vi "SelectOPCTags.RecurseThroughCurrent.vi"(8 "error in (no error)":errorcluster, 9 "Parent":string, 10 "Node Pointer":u64[](array[numeric]) format="%.0x", 11 "Tree":refnum<vi>) -> (0 "error out":errorcluster, 3 "Tree Out":refnum<vi>)   [LabVIEW 2019, in "OPC UA Client Addon System Explorer.lvlib"]
uses:
  OPC UA Client Addon System Explorer.lvlib
  <vilib>/NI VeriStand/Custom Device API/Custom Device API.lvlib
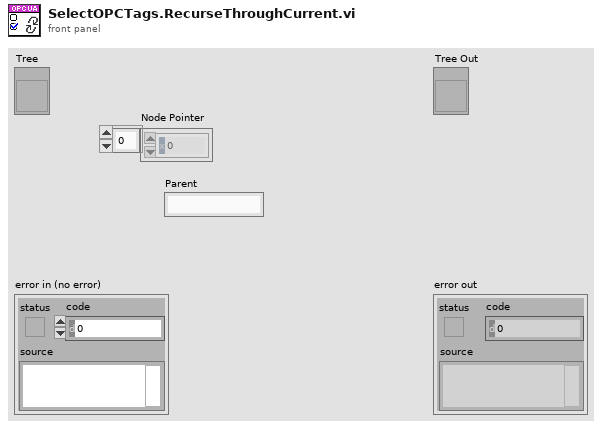
[diagram p1: front panel]
types:
  T1 = typedef "Custom Device API.lvlib/Custom Device Item Info.ctl" = cluster{"Name":string, "Is Channel":bool, "GUID":string, "Is Waveform":bool}
  T2 = typedef "Custom Device API.lvlib/Custom Device Item Ref.ctl" = u64
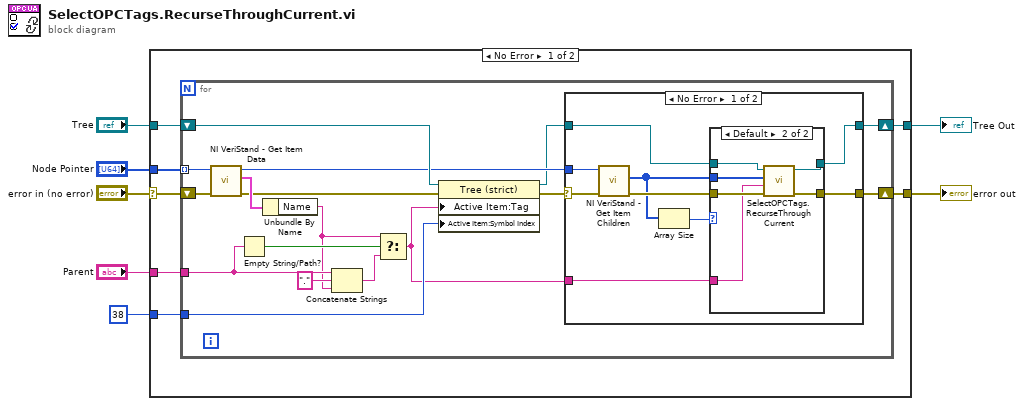
[diagram p0: block diagram]
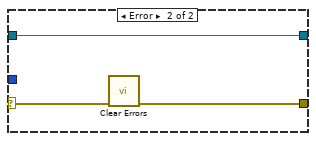
[diagram p3: hidden frame]
diagram:
  n1 = case shown="No Error" "error in (no error)" {
    selector: "error in (no error)" -> [w14 w53]
    tunnel: [w13 w53] -> w6
    tunnel: "Tree" -> [w11 w52]
    tunnel: [w12 w52] -> w4
    tunnel: 38 ("Symbol Index (38)") -> [w10 _]
    tunnel: "Node Pointer" -> [w9 _]
    tunnel: "Parent" -> [w8 _]
    frame No Error {
      n2 = for {
        tunnel: w10 -> [w30]
        shift-right: [w23] -> w13
        shift-left: w14 -> [w29]
        shift-right: [w21] -> w12
        shift-left: w11 -> [w31]
        tunnel: w9 -> [w28] mode=indexing
        tunnel: w8 -> [w20]
        n3 = call <vilib>:"NI VeriStand - Get Item Data.vi"("error in (no error)"=w29, "Item Ref in"=w28) -> ("error out"=w26:errorcluster, "Item Info"=w27:T1, "Item Ref out"=w24:T2)  [unwired: 6 in, 1 out]
        n4 = Empty String/Path?(string/path=w20) -> (empty?=w19:bool)
        n5 = Unbundle By Name(w27) -> ("Name"=w18:string)
        n6 = Concatenate Strings(w20, "." ("string"), w18) -> (w17:string)
        n7 = Select(t=w18, s=w19, f=w17) -> (s? t:f=w16:string)
        n8 = property class="Tree (strict)"(reference=w31, error in=w26, "Active Item:Tag"=w16, "Active Item:Symbol Index"=w30) -> (reference out=w22:refnum<vi>, error out=w15:errorcluster)
        n9 = case shown="No Error" w15 {
          selector: w15 -> [w32 w50]
          tunnel: w24 -> [w40 _]
          tunnel: [w38 w49] -> w23
          tunnel: w22 -> [w36 w51]
          tunnel: [w35 w51] -> w21
          tunnel: w16 -> [w33 _]
          frame No Error {
            n10 = call <vilib>:"NI VeriStand - Get Item Children.vi"("error in (no error)"=w32, "Item Ref in"=w40) -> ("error out"=w39:errorcluster, "Child Refs"=w34:T2[])  [unwired: 6 in, 2 out]
            n11 = Array Size(array=w34) -> (size(s)=w37:i32)
            n12 = case shown="Default" w37 {
              tunnel: w39 -> [w42 w48]
              tunnel: [w42 w47] -> w38
              tunnel: w33 -> [_ w46]
              tunnel: w36 -> [w41 w45]
              tunnel: [w41 w44] -> w35
              tunnel: w34 -> [_ w43]
              frame 0 {
              }
              frame Default {
                n13 = call "SelectOPCTags.RecurseThroughCurrent.vi"("error in (no error)"=w48, "Parent"=w46, "Node Pointer"=w43, "Tree"=w45) -> ("error out"=w47:errorcluster, "Tree Out"=w44:refnum<vi>)  [unwired: 6 in]
              }
            }
          }
          frame Error {
            n14 = call <vilib>:"Clear Errors.vi"("error in (no error)"=w50) -> ("error out"=w49:errorcluster)  [unwired: 5 in, 1 out]
          }
        }
      }
    }
    frame Error {
    }
  }
  "error out" <- w6
  "Tree Out" <- w4
